vi "CMN_Rel2AbsPath.vi"(8 "error in (no error)":errorcluster, 10 "test path":path, 11 "absolute path":path) -> (0 "error out":errorcluster, 2 "output path (str)":string, 3 "output path":path)   [LabVIEW 2016]
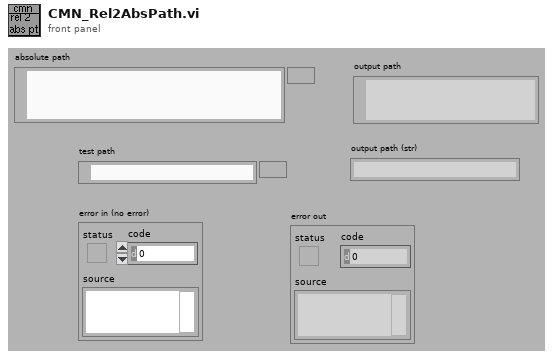
[diagram p1: front panel]
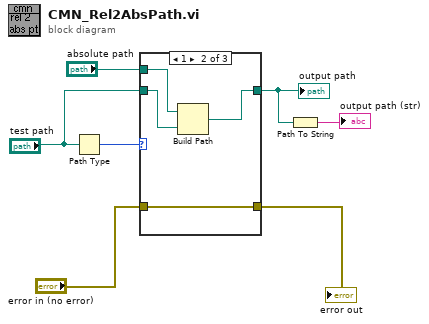
[diagram p0: block diagram]
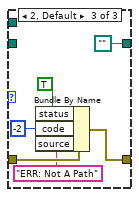
[diagram p3: hidden frame]
diagram:
  n1 = Path Type(1:"test path") -> (0:w7:i16)
  n2 = case shown="1" w7 {
    tunnel: [w9 w11 path ""] -> w5
    tunnel: "test path" -> [w9 w12 _]
    tunnel: "absolute path" -> [_ w13 _]
    tunnel: "error in (no error)" -> [w8 w10 w19]
    tunnel: [w8 w10 w18] -> w1
    frame 0 {
    }
    frame 1 {
      n3 = Build Path(base path=w13, name or relative path=w12) -> (appended path=w11:path)
    }
    frame 2, Default {
      n4 = Bundle By Name(cluster=w19, "status"=TRUE, "code"=-2, "source"="ERR: Not A Path") -> (w18:errorcluster)
    }
  }
  "output path" <- w5
  "error out" <- w1
  n5 = Path To String(path=w5) -> (string=→"output path (str)":string)
